vi "XML Get Acquisition Chassis.vi"(11 "Acquisition Network":T2) -> (1 "Acquisition Chassis Names":string[](array[string]), 2 "Number of BPM Readings":i32, 3 "Acquisition Variable Names":string[][](array[string]), 4 "Inverse BPM Matrix Mapping":u32[][](array[numeric]), 5 "BPM Parameters":T1[](array[typedef]), 6 "BPM Matrix Mapping":cluster{u32[]}[](array[cluster]), 7 "Selected BPM Readings":u32[](array[numeric]))   [LabVIEW 2011, in "XML VIs.lvlib"]
doc: "Extracts the Acquisition Network configuration data (ordered by chassis-by-chassis) and builds dedicated clusters for each configuration (ordered by response matrix row indexes)."
uses:
  XML VIs.lvlib
  Types Definitions/Type Acquisition Network Configuration.ctl
  Types Definitions/Type BPM Parameters.ctl
  Type Definitions.lvlib
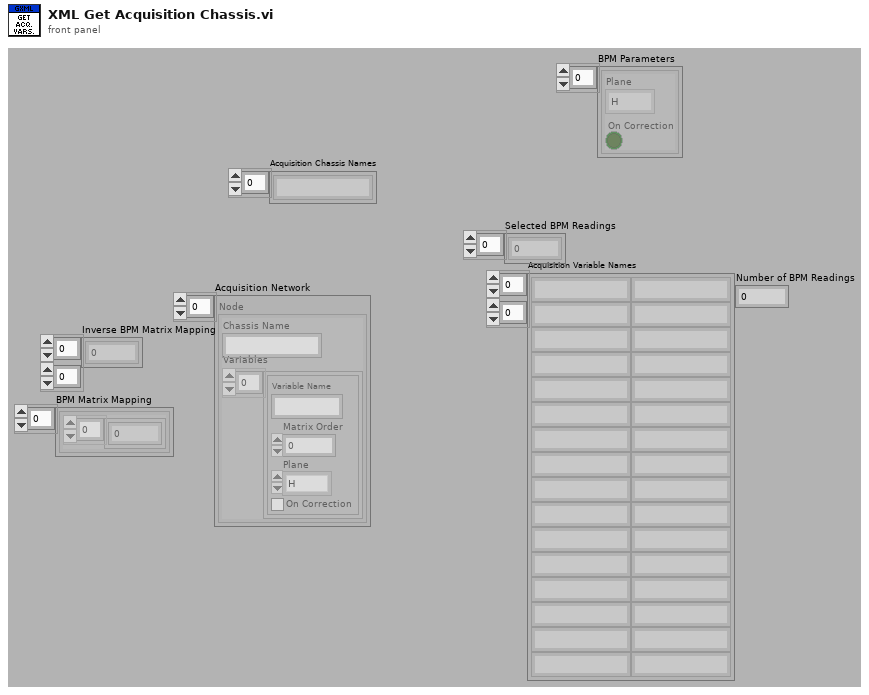
[diagram p1: front panel]
types:
  T1 = typedef "Type Definitions.lvlib/Type BPM Parameters.ctl" = cluster{"Plane":enum8{"H", "V"}, "On Correction":bool}
  T2 = typedef "Type Definitions.lvlib/Type Acquisition Network Configuration.ctl" = cluster{"Chassis Name":string, "Variables":cluster{"Variable Name":string, "Matrix Order":u32, "Plane":enum8{"H", "V"}, "On Correction":bool}[]}[]
  T3 = cluster{"Variable Name":string, "Matrix Order":u32, "Plane":enum8{"H", "V"}, "On Correction":bool}[]
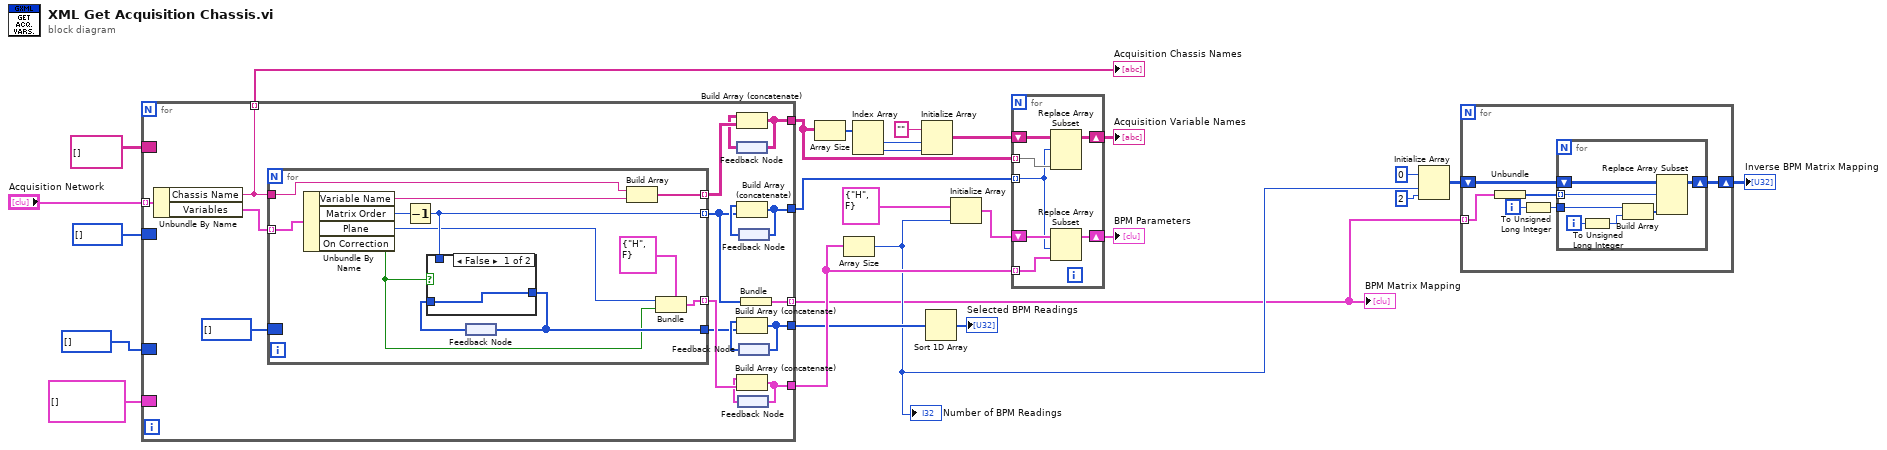
[diagram p0: block diagram]
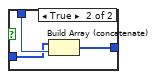
[diagram p2: hidden frame]
diagram:
  n1 = for {
    tunnel: "Acquisition Network" -> [w43] mode=indexing
    tunnel: [w39] -> w18 mode=indexing
    tunnel: [w30] -> w8
    tunnel: [w36] -> w13
    border: T1[] [] -> [_]
    border: u32[] [] -> [_]
    border: string[][] [] -> [_]
    tunnel: [w33] -> w11
    tunnel: [w32] -> w10
    border: u32[] [] -> [_]
    tunnel: [w27] -> w1 mode=indexing
    n2 = Unbundle By Name(w43) -> ("Chassis Name"=w39:string, "Variables"=w42:T3)
    n3 = for {
      tunnel: w42 -> [w55] mode=indexing
      tunnel: w39 -> [w53]
      tunnel: [w48] -> w28 mode=indexing
      tunnel: [w52] -> w41 mode=indexing
      tunnel: [w49] -> w38 mode=indexing
      tunnel: [w46] -> w29
      border: u32[] [] -> [_]
      n4 = Unbundle By Name(w55) -> ("Variable Name"=w54:string, "Matrix Order"=w51:u32, "Plane"=w45:enum8{"H", "V"}, "On Correction"=w44:bool)
      n5 = Decrement(x=w51) -> (x-1=w48:u32)
      n6 = feedback #1() -> (w47:u32[])
      n7 = case shown="False" w44 {
        tunnel: w48 -> [_ w59]
        tunnel: w47 -> [w56 w58]
        tunnel: [w56 w57] -> w46
        frame False {
        }
        frame True {
          n8 = Build Array (concatenate)(w58, w59) -> (w57:u32[])
        }
      }
      n9 = feedback-in #1(w46) -> ()
      n10 = Build Array(w53, w54) -> (w52:string[])
      n11 = Bundle(cluster=T1 {"Plane"=enum."H", "On Correction"=FALSE} ("BPM Parameters"), "Plane"=w45, "On Correction"=w44) -> (w49:T1)
    }
    n12 = feedback #2() -> (w40:string[][])
    n13 = Build Array (concatenate)(w40, w41) -> (w33:string[][])
    n14 = feedback-in #2(w33) -> ()
    n15 = feedback #3() -> (w37:T1[])
    n16 = Build Array (concatenate)(w37, w38) -> (w36:T1[])
    n17 = feedback-in #3(w36) -> ()
    n18 = feedback #4() -> (w34:u32[])
    n19 = Build Array (concatenate)(w34, w28) -> (w32:u32[])
    n20 = feedback-in #4(w32) -> ()
    n21 = feedback #5() -> (w31:u32[])
    n22 = Build Array (concatenate)(w31, w29) -> (w30:u32[])
    n23 = feedback-in #5(w30) -> ()
    n24 = Bundle(w28) -> (w27:cluster{u32[]})  [unwired: 1 in]
  }
  "Acquisition Chassis Names" <- w18
  "BPM Matrix Mapping" <- w1
  n25 = Array Size(array=w11) -> (size(s)=w26:i32[])
  n26 = Array Size(array=w13) -> (size(s)=w2:i32)
  "Number of BPM Readings" <- w2
  n27 = Index Array(array=w26) -> (element #1=w25:i32, element #2=w24:i32)  [unwired: 2 in]
  n28 = Initialize Array("" ("element"), w25, w24) -> (w23:string[][])
  n29 = Sort 1D Array(array=w8) -> (sorted array=→"Selected BPM Readings":u32[])
  n30 = Initialize Array(T1 {"Plane"=enum."H", "On Correction"=FALSE} ("BPM Parameters"), w2) -> (w15:T1[])
  n31 = for {
    shift-right: [w65] -> w21
    shift-left: w23 -> [w66]
    tunnel: w11 -> [w64] mode=indexing
    tunnel: w10 -> [w60] mode=indexing
    shift-right: [w62] -> w14
    shift-left: w15 -> [w63]
    tunnel: w13 -> [w61] mode=indexing
    n32 = Replace Array Subset(array=w66, new element=w64, index (row)=w60) -> (w65:string[][])  [unwired: 1 in]
    n33 = Replace Array Subset(array=w63, new element=w61, index=w60) -> (w62:T1[])
  }
  "Acquisition Variable Names" <- w21
  "BPM Parameters" <- w14
  n34 = Initialize Array(u32 0 ("element"), w2, 2 ("dimension size")) -> (w4:u32[][])
  n35 = for {
    shift-right: [w71] -> w3
    shift-left: w4 -> [w72]
    tunnel: w1 -> [w68] mode=indexing
    i -> [w70]
    n36 = Unbundle(w68) -> (w67:u32[])
    n37 = To Unsigned Long Integer(number=w70) -> (unsigned 32bit integer=w69:u32)
    n38 = for {
      tunnel: w69 -> [w77]
      shift-right: [w78] -> w71
      shift-left: w72 -> [w79]
      tunnel: w67 -> [w75] mode=indexing
      i -> [w73]
      n39 = To Unsigned Long Integer(number=w73) -> (unsigned 32bit integer=w74:u32)
      n40 = Build Array(w77, w74) -> (w76:u32[])
      n41 = Replace Array Subset(array=w79, new element=w76, index (row)=w75) -> (w78:u32[][])  [unwired: 1 in]
    }
  }
  "Inverse BPM Matrix Mapping" <- w3
